vi "Cuboid bounding circle test.vi"(1 "Minimum separation":dbl, 2 "Cuboid 2":T1={"Vertices (x, y)"=[[0.0, 0.0], [0.0, 0.0], [0.0, 0.0], [0.0, 0.0]], "Zmin"=0.0, "Zmax"=0.0, "Centroid (x, y)"=[0.0, 0.0], "Radius"=0.0, "Edge normals (x, y)"=[[0.0, 0.0], [0.0, 0.0], [0.0, 0.0], [0.0, 0.0]], "Edge vectors (x, y)"=[[0.0, 0.0], [0.0, 0.0], [0.0, 0.0], [0.0, 0.0]]}, 3 "Cuboid 1":T1={"Vertices (x, y)"=[[0.0, 0.0], [0.0, 0.0], [0.0, 0.0], [0.0, 0.0]], "Zmin"=0.0, "Zmax"=0.0, "Centroid (x, y)"=[0.0, 0.0], "Radius"=0.0, "Edge normals (x, y)"=[[0.0, 0.0], [0.0, 0.0], [0.0, 0.0], [0.0, 0.0]], "Edge vectors (x, y)"=[[0.0, 0.0], [0.0, 0.0], [0.0, 0.0], [0.0, 0.0]]}) -> (0 "Possible collision":bool)   [LabVIEW 2013]
uses:
  Cuboid properties.ctl
  <vilib>/Analysis/baseanly.llb/Real Dot Product.vi
  <vilib>/Analysis/NI_AALBase.lvlib
panel:
  # "PN 30/08/2014"
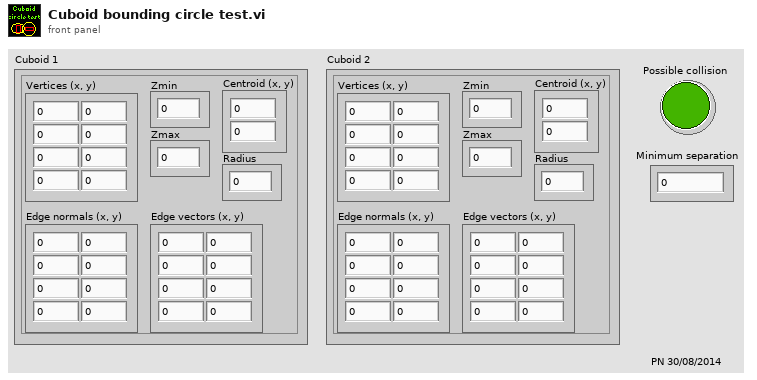
[diagram p1: front panel]
types:
  T1 = typedef "Cuboid properties.ctl" = cluster{"Vertices (x, y)":dbl[][], "Zmin":dbl, "Zmax":dbl, "Centroid (x, y)":dbl[], "Radius":dbl, "Edge normals (x, y)":dbl[][], "Edge vectors (x, y)":dbl[][]}
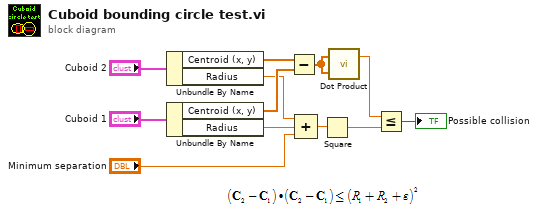
[diagram p0: block diagram]
diagram:
  n1 = Unbundle By Name("Cuboid 2") -> ("Centroid (x, y)"=w10:dbl[], "Radius"=w7:dbl)
  n2 = Unbundle By Name("Cuboid 1") -> ("Centroid (x, y)"=w9:dbl[], "Radius"=w6:dbl)
  n3 = Subtract(x=w10, y=w9) -> (x-y=w8:dbl[])
  n4 = Compound Arithmetic op=ADD(w7, w6, "Minimum separation") -> (w4:dbl)
  n5 = Square(x=w4) -> (x^2=w3:dbl)
  n6 = call-poly <vilib>:"Dot Product.vi"("Y Vector"=w8, "X Vector"=w8) -> ("X * Y"=w2:dbl)  [unwired: 1 out]
  n7 = Less Or Equal?(x=w2, y=w3) -> (x <= y?=→"Possible collision":bool)
